vi "switches_builder.vi"(7 "measure?":dbl, 11 "Switches data":path) -> (3 "closed switches (out)":string)   [LabVIEW 2020]
uses:
  <vilib>/Utility/file.llb/Read From Spreadsheet File (DBL).vi
panel:
  out "chaves fechadas":dbl[][](array[numeric])
  # "SWITCHES BUILDER"
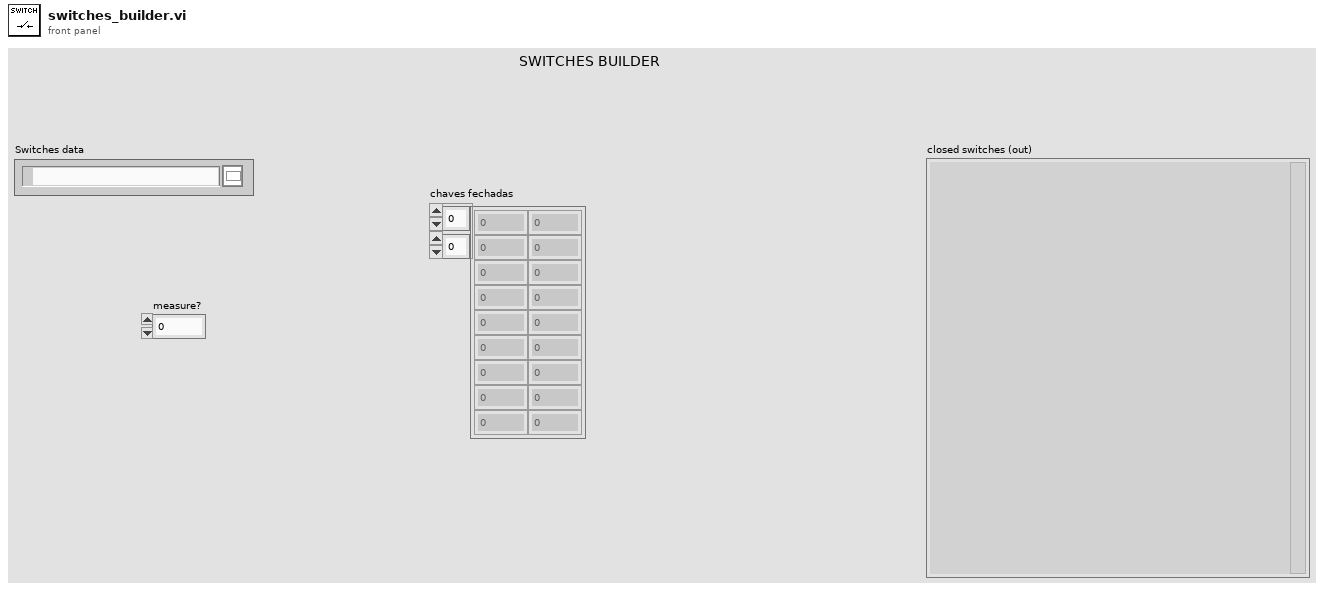
[diagram p1: front panel]
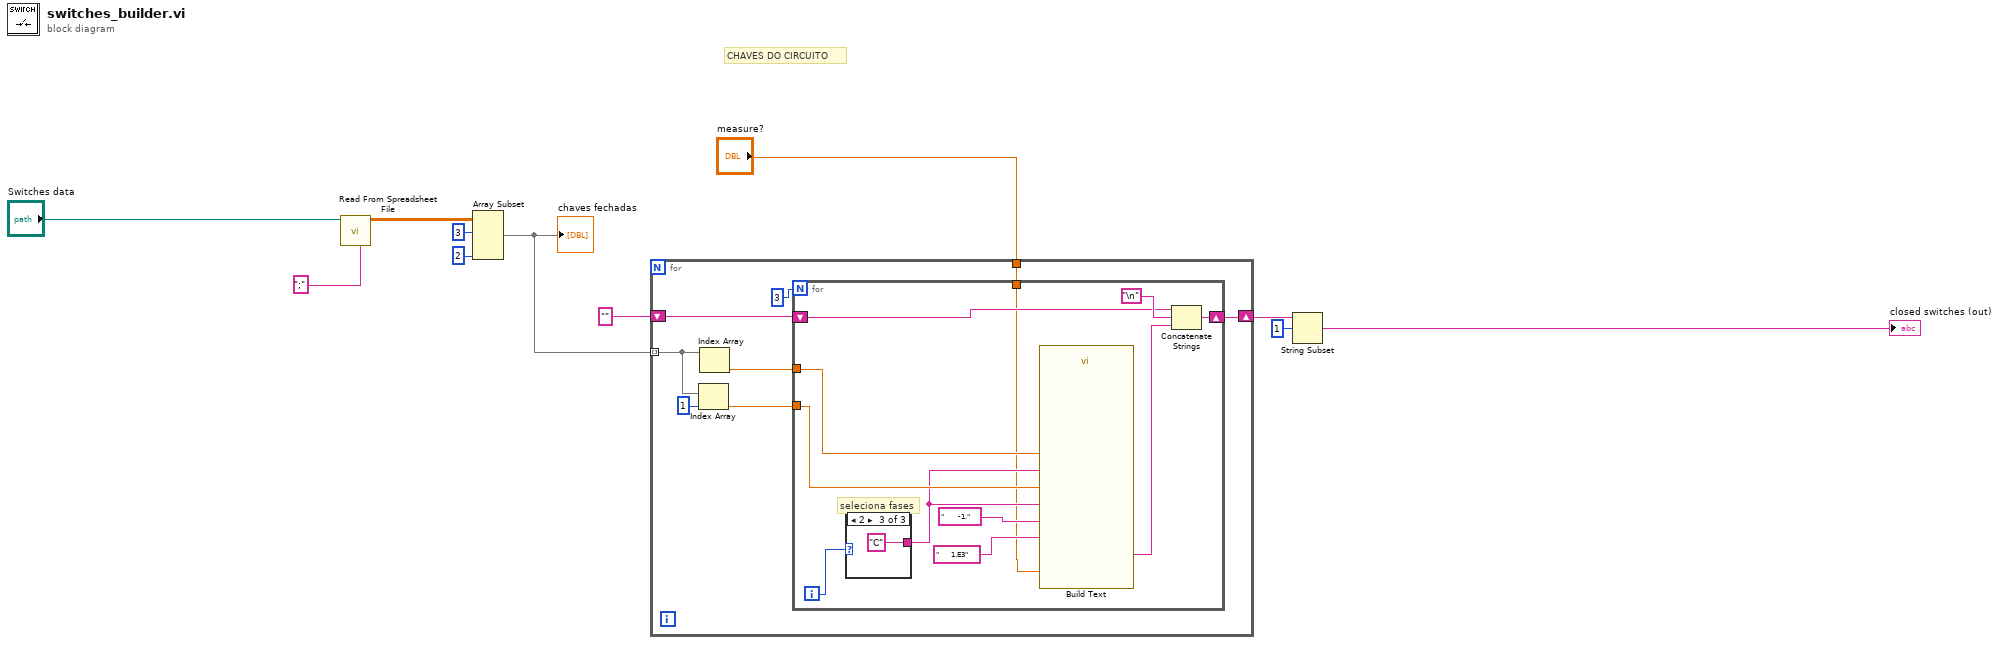
[diagram p0: block diagram]
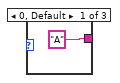
[diagram p2: hidden frame]
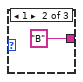
[diagram p3: hidden frame]
diagram:
  # "CHAVES DO CIRCUITO"
  n1 = call-poly <vilib>:"Read From Spreadsheet File.vi"("delimiter (\\t)"=";" ("delimiter (\\t)"), "file path (dialog if empty)"="Switches data") -> ("all rows"=w10:dbl[][])  [unwired: 5 in, 4 out]
  n2 = Array Subset(array=w10, index (row)=3 ("index"), length (col)=2 ("length")) -> (w7:dbl[][])  [unwired: 2 in]
  "chaves fechadas" <- w7
  n3 = for {
    tunnel: w7 -> [w19] mode=indexing
    shift-right: [w16] -> w4
    shift-left: "" -> [w17]
    tunnel: "measure?" -> [w12]
    n4 = Index Array(array=w19, index=1) -> (element=w14:dbl)
    n5 = Index Array(array=w19) -> (element=w15:dbl)  [unwired: 1 in]
    n6 = for {
      N: 3 -> [_]
      shift-right: [w30] -> w16
      shift-left: w17 -> [w21]
      tunnel: w15 -> [w29]
      tunnel: w14 -> [w28]
      tunnel: w12 -> [w20]
      i -> [w27]
      # "seleciona fases"
      n7 = case shown="2" w27 {
        tunnel: ["A" "B" "C"] -> w26
        frame 0, Default {
        }
        frame 1 {
        }
        frame 2 {
        }
      }
      n8 = call "Build Text"("fase_out"=w26, "Topen"="      1.E3", "de"=w29, "fase_in"=w26, "para"=w28, "Tclose"="       -1.", "measure"=w20) -> ("Result"=w23:string)  [unwired: 7 in, 1 out]
      n9 = Concatenate Strings(w21, "\n", w23) -> (w30:string)
    }
  }
  n10 = String Subset(string=w4, offset (0)=1) -> (substring=→"closed switches (out)":string)  [unwired: 1 in]
